vi "Read Calibration Result.vi"(8 "error in (no error)":errorcluster, 11 "VISA resource name":refnum<visa-resource-name>) -> (0 "error out":errorcluster, 1 "Time":string, 2 "Date":string, 3 "VISA resource name out":refnum<visa-resource-name>, 4 "Temperature":string, 5 "Status":string)   [LabVIEW 2015, in "Agilent 2000 3000 X-Series.lvlib"]
doc: "Returns the calibration result."
uses:
  <instrlib>/Agilent 2000 3000 X-Series/Agilent 2000 3000 X-Series.lvlib
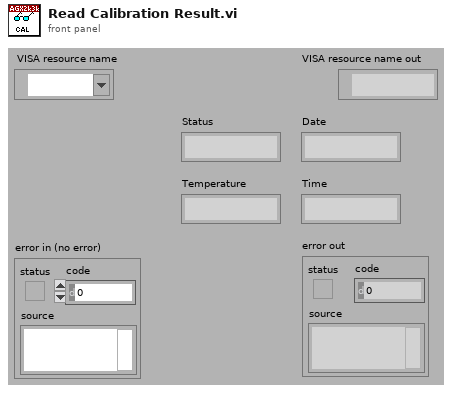
[diagram p1: front panel]
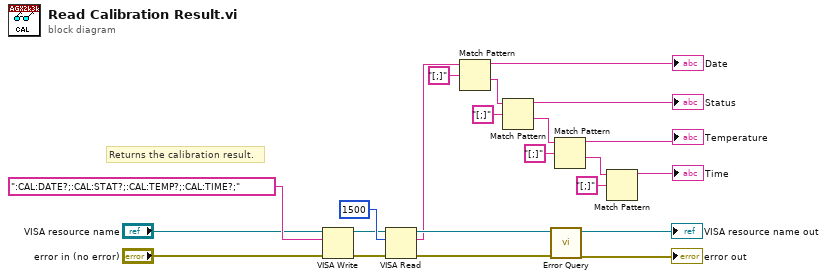
[diagram p0: block diagram]
diagram:
  # "Returns the calibration result."
  n1 = VISA Write(VISA resource name="VISA resource name", write buffer=":CAL:DATE?;:CAL:STAT?;:CAL:TEMP?;:CAL:TIME?;", error in (no error)="error in (no error)") -> (VISA resource name out=w8:refnum<visa-resource-name>, error out=w9:errorcluster)  [unwired: 1 out]
  n2 = VISA Read(VISA resource name=w8, byte count=u32 1500, error in (no error)=w9) -> (VISA resource name out=w7:refnum<visa-resource-name>, read buffer=w5:string, error out=w6:errorcluster)  [unwired: 1 out]
  n3 = Match Pattern(string=w5, regular expression="[;]") -> (before substring=→"Date":string, after substring=w13:string)  [unwired: 3 out]
  n4 = Match Pattern(string=w13, regular expression="[;]") -> (before substring=→"Status":string, after substring=w12:string)  [unwired: 3 out]
  n5 = call <instrlib>:"Error Query.vi"("error in (no error)"=w6, "VISA resource name"=w7) -> ("error out"=→"error out":errorcluster, "VISA resource name out"=→"VISA resource name out":refnum<visa-resource-name>)  [unwired: 8 out]
  n6 = Match Pattern(string=w12, regular expression="[;]") -> (before substring=→"Temperature":string, after substring=w11:string)  [unwired: 3 out]
  n7 = Match Pattern(string=w11, regular expression="[;]") -> (before substring=→"Time":string)  [unwired: 4 out]
